vi "TCP Send Packet.vi"(8 "error in (no error)":errorcluster, 10 "TCPPacket":refnum<class "TCPPacket.lvclass">, 11 "TCP Refnum In":refnum<k5>) -> (0 "error out":errorcluster, 3 "TCP Refnum Out":refnum<k5>)   [LabVIEW 2019]
uses:
  TCPPacket/TCPPacket.lvclass
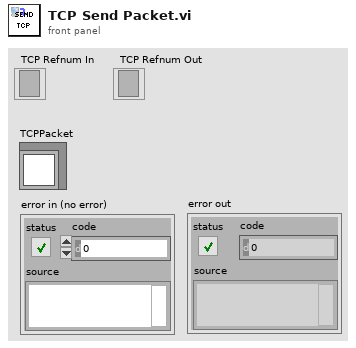
[diagram p1: front panel]
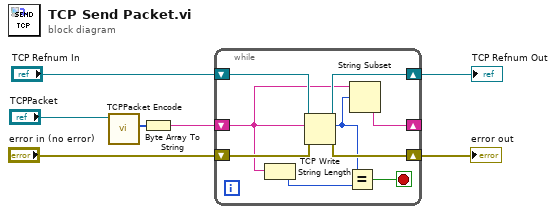
[diagram p0: block diagram]
diagram:
  n1 = call-dynamic "TCPPacket Encode.vi"("TCPPacket in"="TCPPacket") -> ("Data"=w6:u8[])  [unwired: 8 in, 2 out]
  n2 = Byte Array To String(unsigned byte array=w6) -> (string=w1:string)
  n3 = while {
    shift-right: [w15] -> w4
    shift-left: "TCP Refnum In" -> [w16]
    shift-right: [w13] -> w2
    shift-left: "error in (no error)" -> [w14]
    shift-right: [w8] -> _
    shift-left: w1 -> [w10]
    stop <- w12 stop-if-true
    n4 = String Length(string=w10) -> (length=w11:i32)
    n5 = TCP Write(connection ID=w16, data in=w10, error in (no error)=w14) -> (connection ID out=w15:refnum<k5>, bytes written=w9:i32, error out=w13:errorcluster)  [unwired: 1 in]
    n6 = Equal?(x=w9, y=w11) -> (x = y?=w12:bool)
    n7 = String Subset(string=w10, offset (0)=w9) -> (substring=w8:string)  [unwired: 1 in]
  }
  "TCP Refnum Out" <- w4
  "error out" <- w2
